vi "Read Tag Disconnect Behavior.vi"(8 "error in (no error)":errorcluster, 11 "CIFChannels in":refnum<class "CIFChannels.lvclass">) -> (0 "error out":errorcluster, 2 "Disconnect Behavior":T1, 3 "CIFChannels out":refnum<class "CIFChannels.lvclass">)   [LabVIEW 2021, in "CIFChannels.lvclass"]
uses:
  CIFChannels.lvclass
  ChannelCommon/typedef/Disconnect Behavior.ctl
  CIFChannels.lvclass/CIFChannels.ctl
  ChannelCommon/ChannelCommon.lvlib
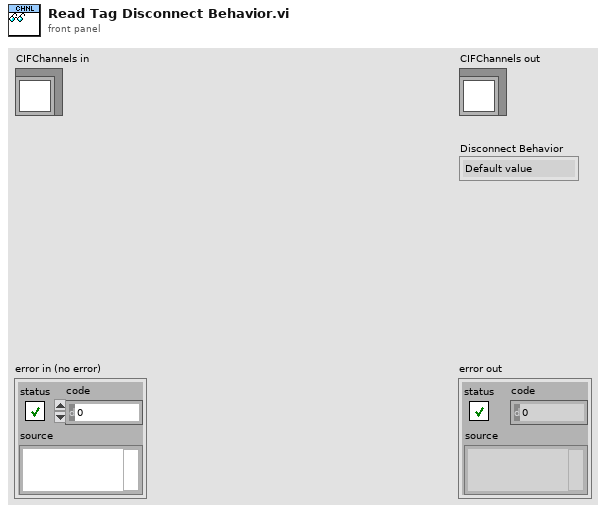
[diagram p1: front panel]
types:
  T1 = typedef "ChannelCommon.lvlib/Disconnect Behavior.ctl" = enum8{"Default value", "Last value", "Error with default"}
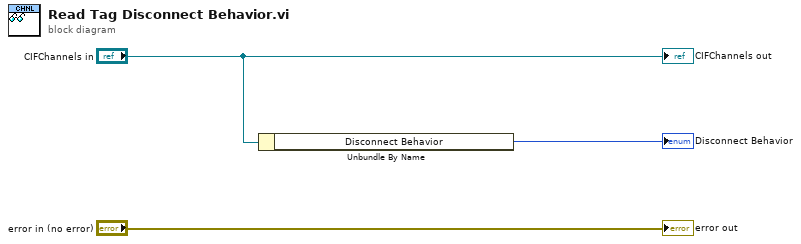
[diagram p0: block diagram]
diagram:
  n1 = Unbundle By Name("CIFChannels in") -> ("Disconnect Behavior"=→"Disconnect Behavior":T1)
  "error out" <- "error in (no error)"
  "CIFChannels out" <- "CIFChannels in"
